vi "DragandDrop.vi"() -> ()   [LabVIEW 2023]
uses:
  <vilib>/picture/picture.llb/imagedata.ctl
panel:
  out "output cluster 3":T1
  out "output cluster 2":T1
  out "np 4":picture
  out "output cluster":T1
  in  "Resi":bool
  in  "Conde":bool
  in  "Bobi":bool
  out "Resi indi":bool
  in  "R":path
  out "Conde indi":bool
  in  "C":path
  out "Bobi indi":bool
  in  "stop 3":bool
  in  "L":path
  in  "stop":bool
  out "Arrastrar boton":bool
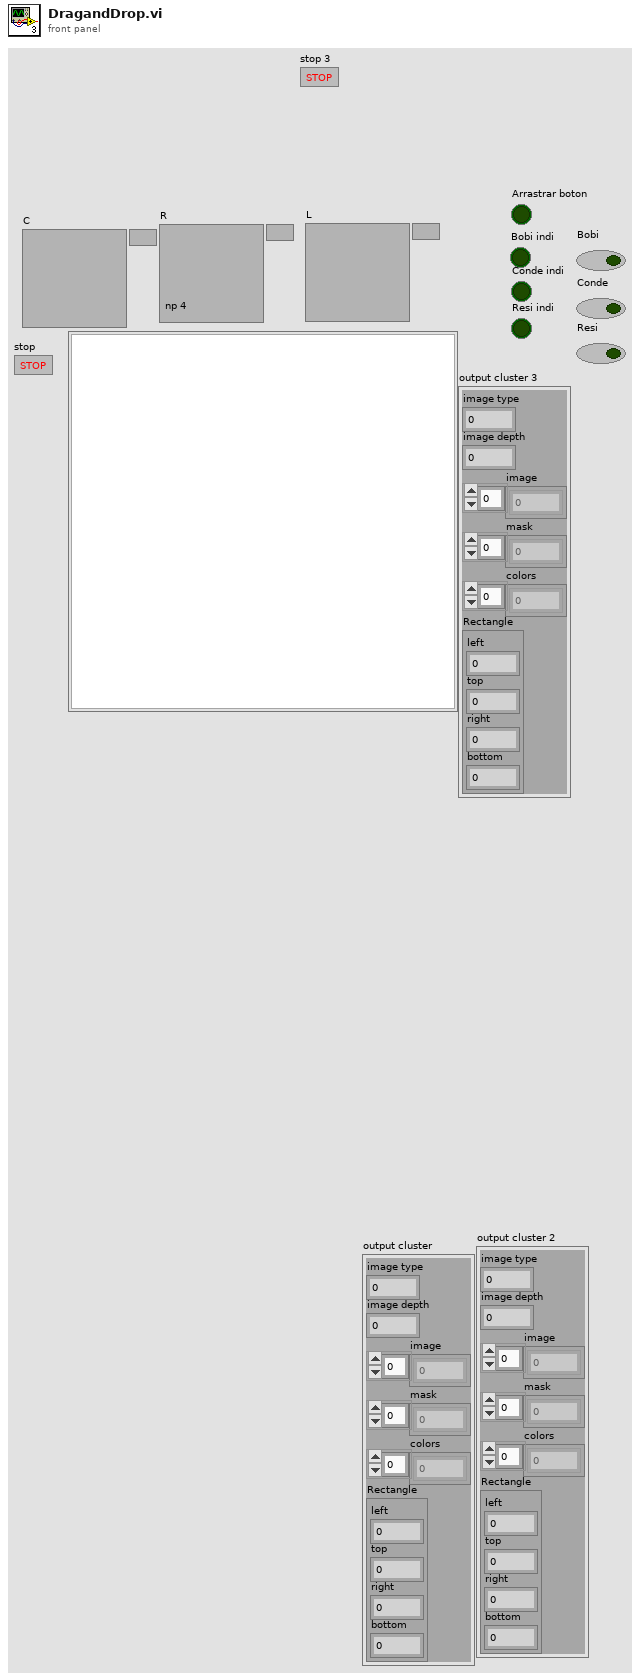
[diagram p1: front panel]
types:
  T1 = typedef "imagedata.ctl" = cluster{"image type":i32, "image depth":i32, "image":u8[], "mask":u8[], "colors":u32[], "Rectangle":cluster{"left":i16, "top":i16, "right":i16, "bottom":i16}}
  T2 = typedef "LVPoint32TypeDef.ctl" = cluster{"Horizontal":i32, "Vertical":i32}
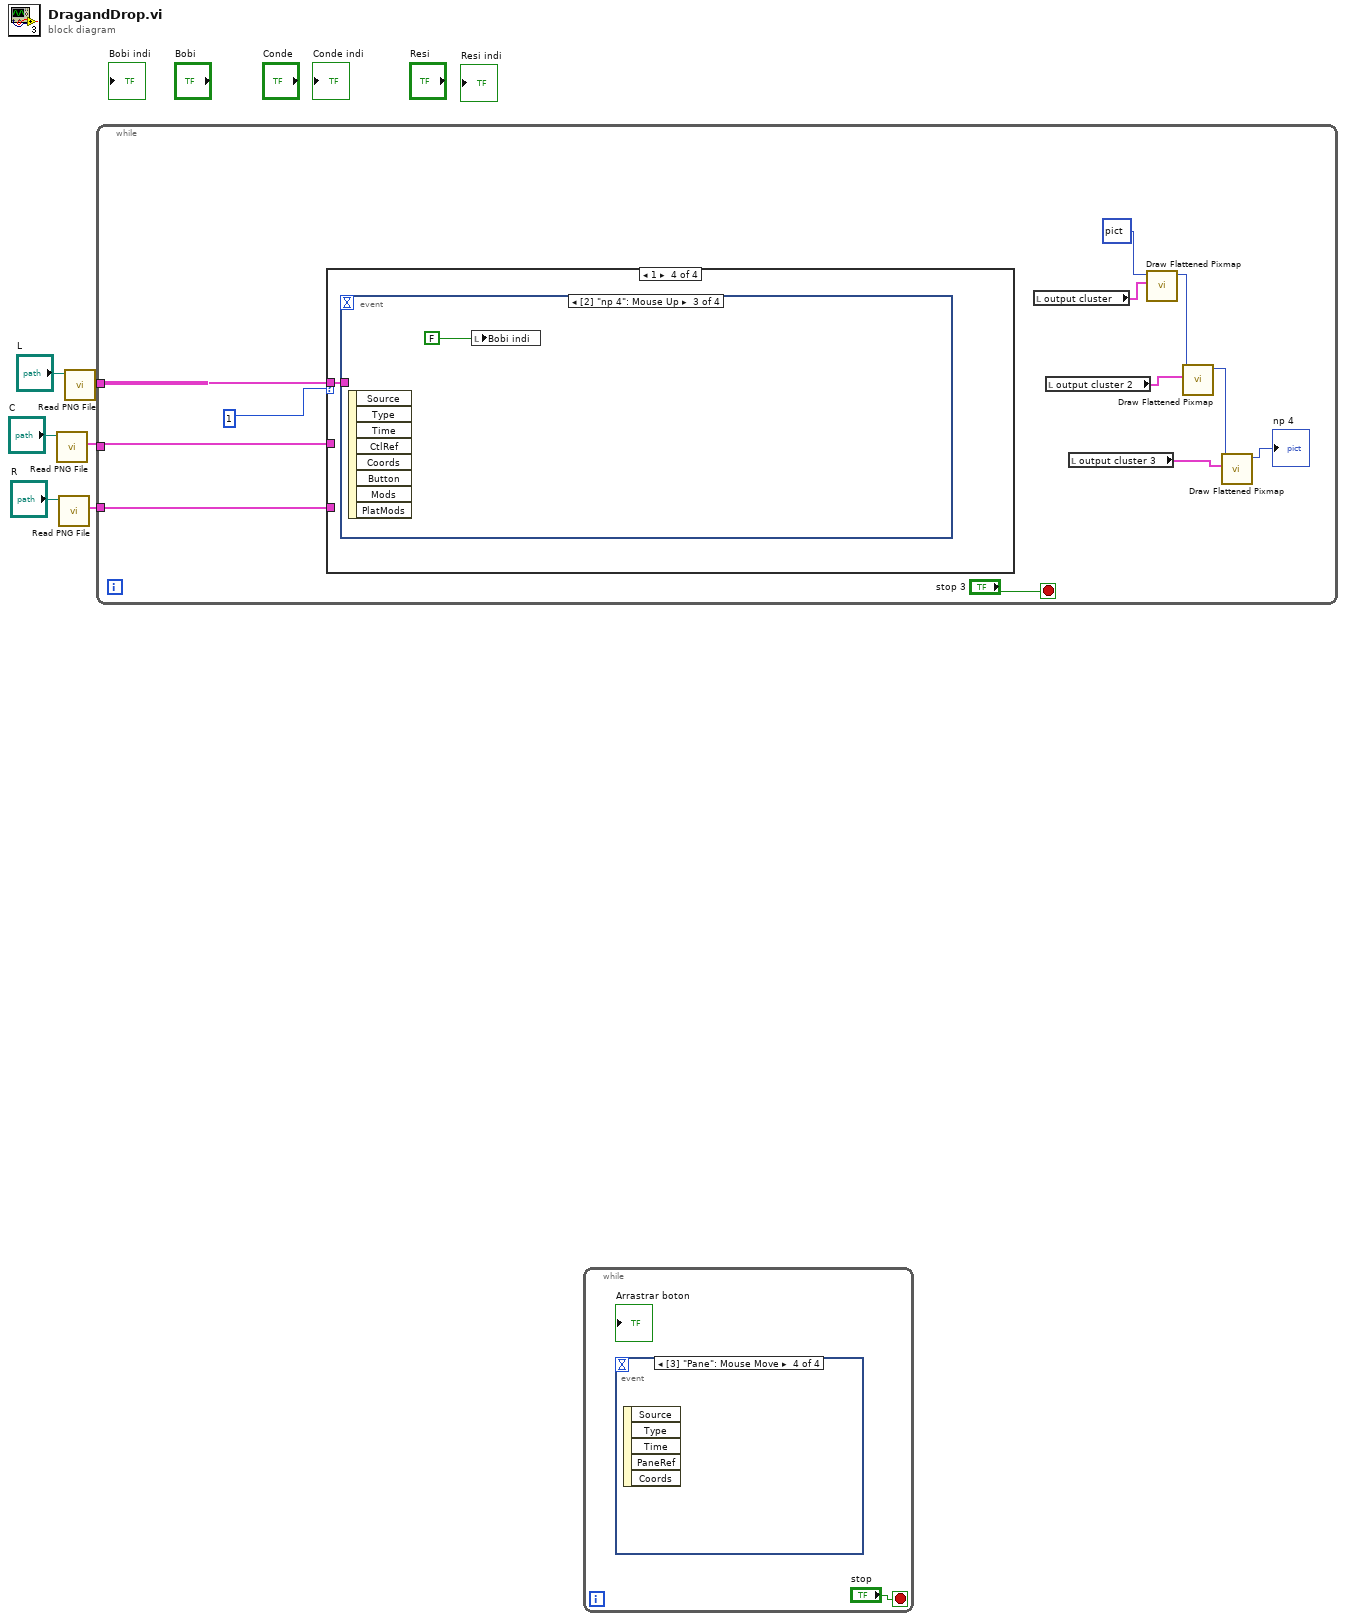
[diagram p0: block diagram]
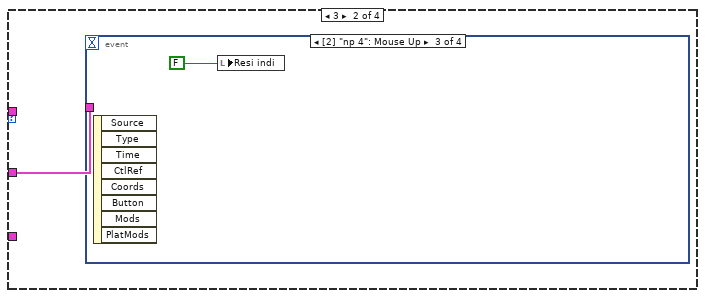
[diagram p3: hidden frame]
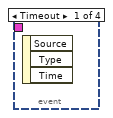
[diagram p4: hidden frame]
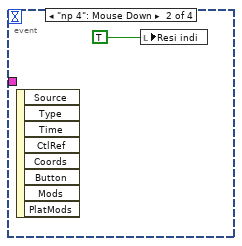
[diagram p5: hidden frame]
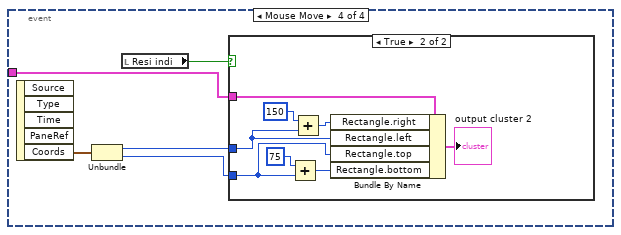
[diagram p6: hidden frame]
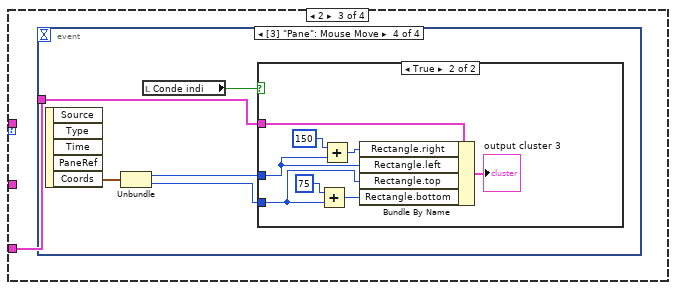
[diagram p8: hidden frame]
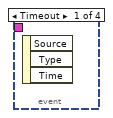
[diagram p9: hidden frame]
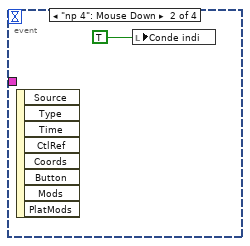
[diagram p10: hidden frame]
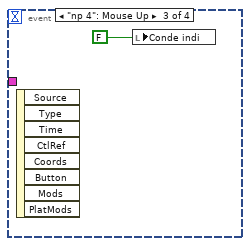
[diagram p11: hidden frame]
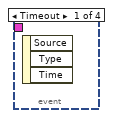
[diagram p13: hidden frame]
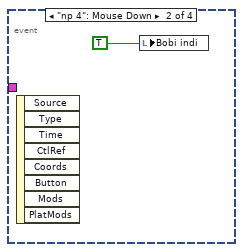
[diagram p14: hidden frame]
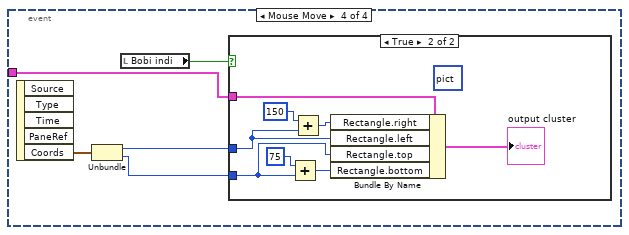
[diagram p15: hidden frame]
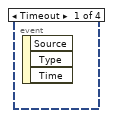
[diagram p17: hidden frame]
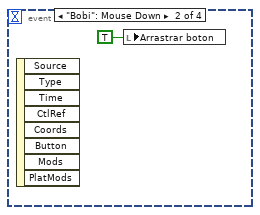
[diagram p18: hidden frame]
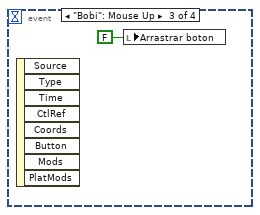
[diagram p19: hidden frame]
diagram:
  n1 = call <vilib>:"Read PNG File.vi"("path to PNG file"="C") -> ("image data"=w3:T1)  [unwired: 8 in, 2 out]
  n2 = call <vilib>:"Read PNG File.vi"("path to PNG file"="R") -> ("image data"=w1:T1)  [unwired: 8 in, 2 out]
  n3 = call <vilib>:"Read PNG File.vi"("path to PNG file"="L") -> ("image data"=w5:T1)  [unwired: 8 in, 2 out]
  n4 = while {
    tunnel: w5 -> [w16]
    tunnel: w3 -> [w17]
    tunnel: w1 -> [w15]
    stop <- "stop 3" stop-if-true
    n5 = case shown="1" 1 {
      tunnel: w16 -> [_ _ _ w51]
      tunnel: w17 -> [_ w19 _ _]
      tunnel: w15 -> [_ _ w35 _]
      frame 0, Default {
      }
      frame 3 {
        n6 = event shown="[2] \"np 4\": Mouse Up" {
          selector: _ -> [_ _ _ _]
          dyn-events: _ -> [_ _ _ _]
          timeout: _ -> [_ _ _ _]
          tunnel: w19 -> [_ _ _ w26]
          event Timeout {
            n7 = event-data() -> ()  [unwired: 1 in, 3 out]
          }
          event "np 4": Mouse Down {
            n8 = event-data() -> ()  [unwired: 1 in, 8 out]
            n9 = local write "Resi indi"(TRUE ("Boolean 2")) -> ()
          }
          event "np 4": Mouse Up {
            n10 = event-data() -> ()  [unwired: 1 in, 8 out]
            n11 = local write "Resi indi"(FALSE ("Arrastrar boton")) -> ()
          }
          event Mouse Move {
            n12 = event-data() -> ("Coords"=w22:T2)  [unwired: 1 in, 4 out]
            n13 = Unbundle(w22) -> ("Horizontal"=w24:i32, "Vertical"=w23:i32)
            n14 = local read "Resi indi"() -> (w25:bool)
            n15 = case shown="True" w25 {
              tunnel: w23 -> [_ w32]
              tunnel: w24 -> [_ w31]
              tunnel: w26 -> [_ w28]
              frame False {
              }
              frame True {
                n16 = Add(x=75 ("Horizontal"), y=w32) -> (x+y=w34:i32)
                n17 = Add(x=150 ("Horizontal"), y=w31) -> (x+y=w33:i32)
                n18 = Bundle By Name(cluster=w28, "Rectangle.right"=w33, "Rectangle.left"=w31, "Rectangle.top"=w32, "Rectangle.bottom"=w34) -> (→"output cluster 2":T1)
              }
            }
          }
        }
      }
      frame 2 {
        n19 = event shown="[3] \"Pane\": Mouse Move" {
          selector: _ -> [_ _ _ _]
          dyn-events: _ -> [_ _ _ _]
          timeout: _ -> [_ _ _ _]
          tunnel: w35 -> [_ _ _ w42]
          event Timeout {
            n20 = event-data() -> ()  [unwired: 1 in, 3 out]
          }
          event "np 4": Mouse Down {
            n21 = event-data() -> ()  [unwired: 1 in, 8 out]
            n22 = local write "Conde indi"(TRUE ("Boolean 2")) -> ()
          }
          event "np 4": Mouse Up {
            n23 = event-data() -> ()  [unwired: 1 in, 8 out]
            n24 = local write "Conde indi"(FALSE ("Arrastrar boton")) -> ()
          }
          event Mouse Move {
            n25 = event-data() -> ("Coords"=w38:T2)  [unwired: 1 in, 4 out]
            n26 = Unbundle(w38) -> ("Horizontal"=w40:i32, "Vertical"=w39:i32)
            n27 = local read "Conde indi"() -> (w41:bool)
            n28 = case shown="True" w41 {
              tunnel: w39 -> [_ w48]
              tunnel: w40 -> [_ w47]
              tunnel: w42 -> [_ w44]
              frame False {
              }
              frame True {
                n29 = Add(x=75 ("Horizontal"), y=w48) -> (x+y=w50:i32)
                n30 = Add(x=150 ("Horizontal"), y=w47) -> (x+y=w49:i32)
                n31 = Bundle By Name(cluster=w44, "Rectangle.right"=w49, "Rectangle.left"=w47, "Rectangle.top"=w48, "Rectangle.bottom"=w50) -> (→"output cluster 3":T1)
              }
            }
          }
        }
      }
      frame 1 {
        n32 = event shown="[2] \"np 4\": Mouse Up" {
          selector: _ -> [_ _ _ _]
          dyn-events: _ -> [_ _ _ _]
          timeout: _ -> [_ _ _ _]
          tunnel: w51 -> [_ _ _ w58]
          event Timeout {
            n33 = event-data() -> ()  [unwired: 1 in, 3 out]
          }
          event "np 4": Mouse Down {
            n34 = event-data() -> ()  [unwired: 1 in, 8 out]
            n35 = local write "Bobi indi"(TRUE ("Boolean 2")) -> ()
          }
          event "np 4": Mouse Up {
            n36 = event-data() -> ()  [unwired: 1 in, 8 out]
            n37 = local write "Bobi indi"(FALSE ("Arrastrar boton")) -> ()
          }
          event Mouse Move {
            n38 = event-data() -> ("Coords"=w54:T2)  [unwired: 1 in, 4 out]
            n39 = Unbundle(w54) -> ("Horizontal"=w56:i32, "Vertical"=w55:i32)
            n40 = local read "Bobi indi"() -> (w57:bool)
            n41 = case shown="True" w57 {
              tunnel: w55 -> [_ w64]
              tunnel: w56 -> [_ w63]
              tunnel: w58 -> [_ w60]
              frame False {
              }
              frame True {
                (unwired) picture data[5B] ("picture")
                n42 = Add(x=75 ("Horizontal"), y=w64) -> (x+y=w66:i32)
                n43 = Add(x=150 ("Horizontal"), y=w63) -> (x+y=w65:i32)
                n44 = Bundle By Name(cluster=w60, "Rectangle.right"=w65, "Rectangle.left"=w63, "Rectangle.top"=w64, "Rectangle.bottom"=w66) -> (→"output cluster":T1)
              }
            }
          }
        }
      }
    }
    n45 = local read "output cluster"() -> (w12:T1)
    n46 = local read "output cluster 2"() -> (w11:T1)
    n47 = local read "output cluster 3"() -> (w8:T1)
    n48 = call <vilib>:"Draw Flattened Pixmap.vi"("image data"=w12, "picture"=picture data[5B]) -> ("new picture"=w10:picture)  [unwired: 7 in]
    n49 = call <vilib>:"Draw Flattened Pixmap.vi"("image data"=w11, "picture"=w10) -> ("new picture"=w9:picture)  [unwired: 7 in]
    n50 = call <vilib>:"Draw Flattened Pixmap.vi"("image data"=w8, "picture"=w9) -> ("new picture"=→"np 4":picture)  [unwired: 7 in]
  }
  n51 = while {
    stop <- "stop" stop-if-true
    n52 = event shown="[3] \"Pane\": Mouse Move" {
      selector: _ -> [_ _ _ _]
      dyn-events: _ -> [_ _ _ _]
      timeout: _ -> [_ _ _ _]
      event Timeout {
        n53 = event-data() -> ()  [unwired: 1 in, 3 out]
      }
      event "Bobi": Mouse Down {
        n54 = event-data() -> ()  [unwired: 1 in, 8 out]
        n55 = local write "Arrastrar boton"(TRUE ("Boolean 2")) -> ()
      }
      event "Bobi": Mouse Up {
        n56 = event-data() -> ()  [unwired: 1 in, 8 out]
        n57 = local write "Arrastrar boton"(FALSE ("Arrastrar boton")) -> ()
      }
      event Mouse Move {
        n58 = event-data() -> ()  [unwired: 1 in, 5 out]
      }
    }
  }
